vi "Generate U.vi"(7 "SLAM In":T2, 8 "error in (no error)":errorcluster, 10 "XYT":cluster{"X":dbl, "Y":dbl, "Theta":dbl}) -> (0 "error out":errorcluster, 3 "U":T1, 5 "SLAM Out":T2)   [LabVIEW 2009]
uses:
  Controls/SLAM.ctl
  <vilib>/Analysis/Matrix/Datatypes/RealMatrix.ctl
  <vilib>/Analysis/Matrix/NI_Matrix.lvlib
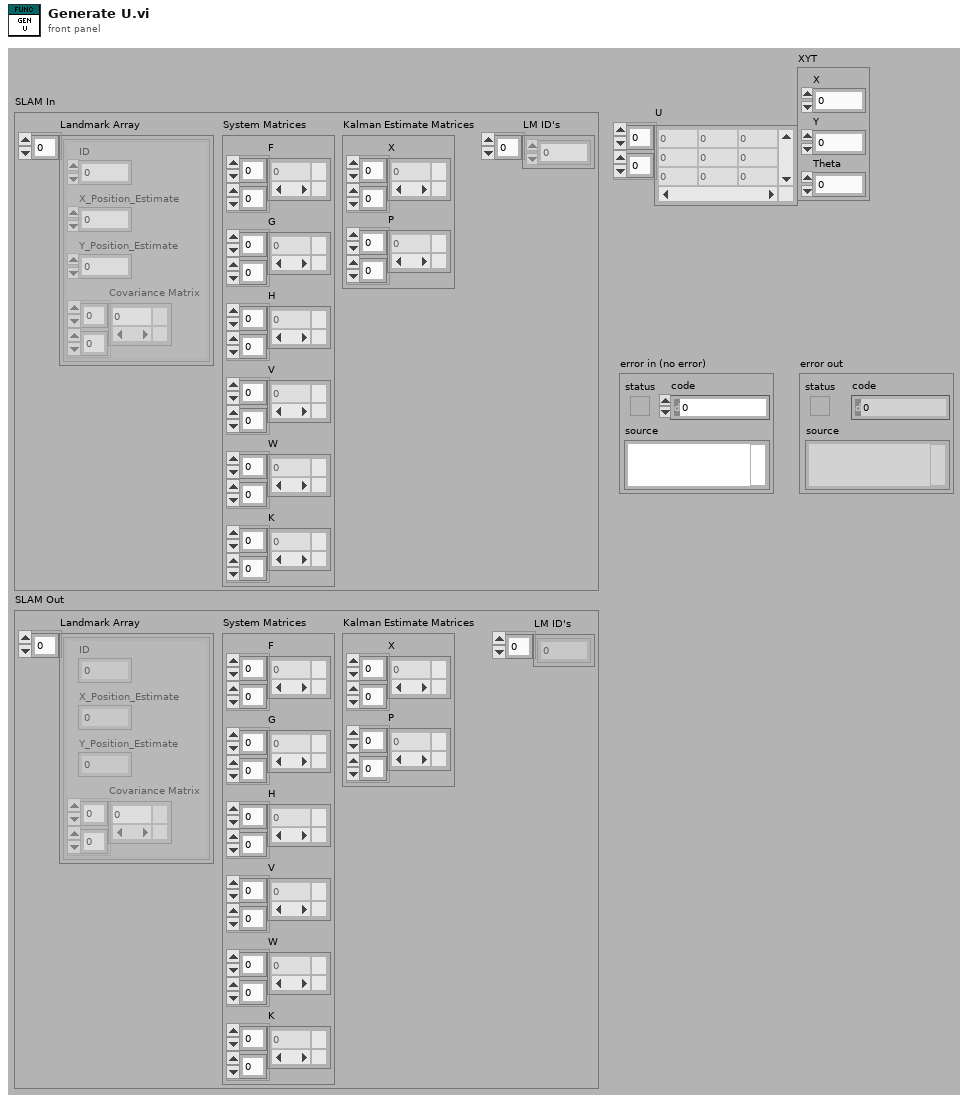
[diagram p1: front panel]
types:
  T1 = typedef "NI_Matrix.lvlib/RealMatrix.ctl" = dbl[][]
  T2 = typedef "SLAM.ctl" = cluster{"Landmark Array":cluster{"ID":dbl, "X_Position_Estimate":dbl, "Y_Position_Estimate":dbl, "Covariance Matrix":T1}[], "System Matrices":cluster{"F":T1, "G":T1, "H":T1, "V":T1, "W":T1, "K":T1}, "Kalman Estimate Matrices":cluster{"X":T1, "P":T1}, "LM ID's":dbl[]}
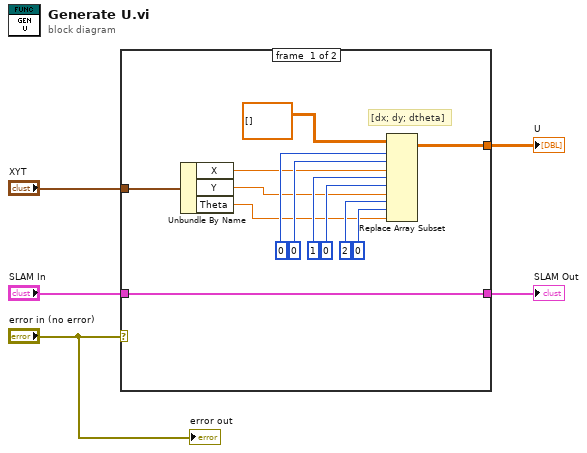
[diagram p0: block diagram]
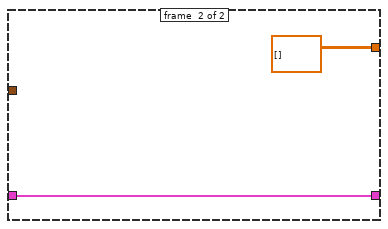
[diagram p2: hidden frame]
diagram:
  n1 = case shown="No Error" "error in (no error)" {
    tunnel: "SLAM In" -> [w8 w20]
    tunnel: [w8 w20] -> w4
    tunnel: [w7 T1 [] ("A x B")] -> w3
    tunnel: "XYT" -> [w11 _]
    frame #0 {
      # "[dx; dy; dtheta]"
      n2 = Unbundle By Name(w11) -> ("X"=w10:dbl, "Y"=w9:dbl, "Theta"=w6:dbl)
      n3 = Replace Array Subset(array=T1 [] ("matrix"), new element #1=w10, index (row) #1=0 ("disabled index (row)"), index (col) #1=0 ("disabled index (row)"), new element #2=w9, index (row) #2=1 ("disabled index (row)"), index (col) #2=0 ("disabled index (row)"), new element #3=w6, index (row) #3=2 ("disabled index (row)"), index (col) #3=0 ("disabled index (row)")) -> (w7:T1)
    }
    frame #1 {
    }
  }
  "SLAM Out" <- w4
  "U" <- w3
  "error out" <- "error in (no error)"
